vi "Set Values.vi"(0 "image in":refnum<class "MSC Image.lvclass">, 1 "imageData U8":u8[][](array[numeric]), 2 "imageData U16":u16[][](array[numeric]), 3 "imageData Single":sgl[][](array[numeric]), 4 "imageData Double":dbl[][](array[numeric]), 5 "error in (no error)":errorcluster, 9 "imageData BGR":u32[][](array[numeric])) -> (14 "image out":refnum<class "MSC Image.lvclass">, 19 "error out":errorcluster)   [LabVIEW 2014, in "MSC Image.lvclass"]
doc: "Sets the values of the image to the connected array values."
uses:
  MSC Image.lvclass
  controls/Image Type.ctl
  MSC Image.lvclass/MSC Image.ctl
  Dependencies/x86/MSC I Process32.dll
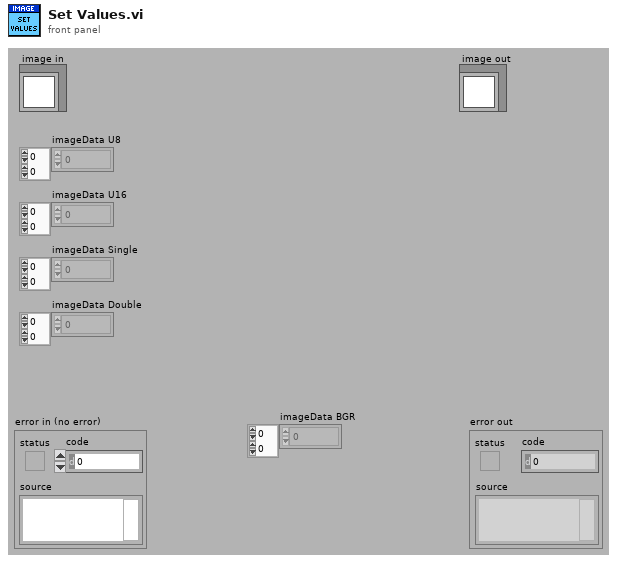
[diagram p1: front panel]
types:
  T1 = typedef "MSC Image.lvclass/Image Type.ctl" = i32
  T2 = typedef "Image.ctl" = cluster{"Pointer":u64, "Size":T3, "Image Type":T4, "Time Stamp":timestamp, "Variant":variant}
  T3 = typedef "Size.ctl" = cluster{"Cols":i32, "Rows":i32}
  T4 = typedef "Image Type.ctl" = i32
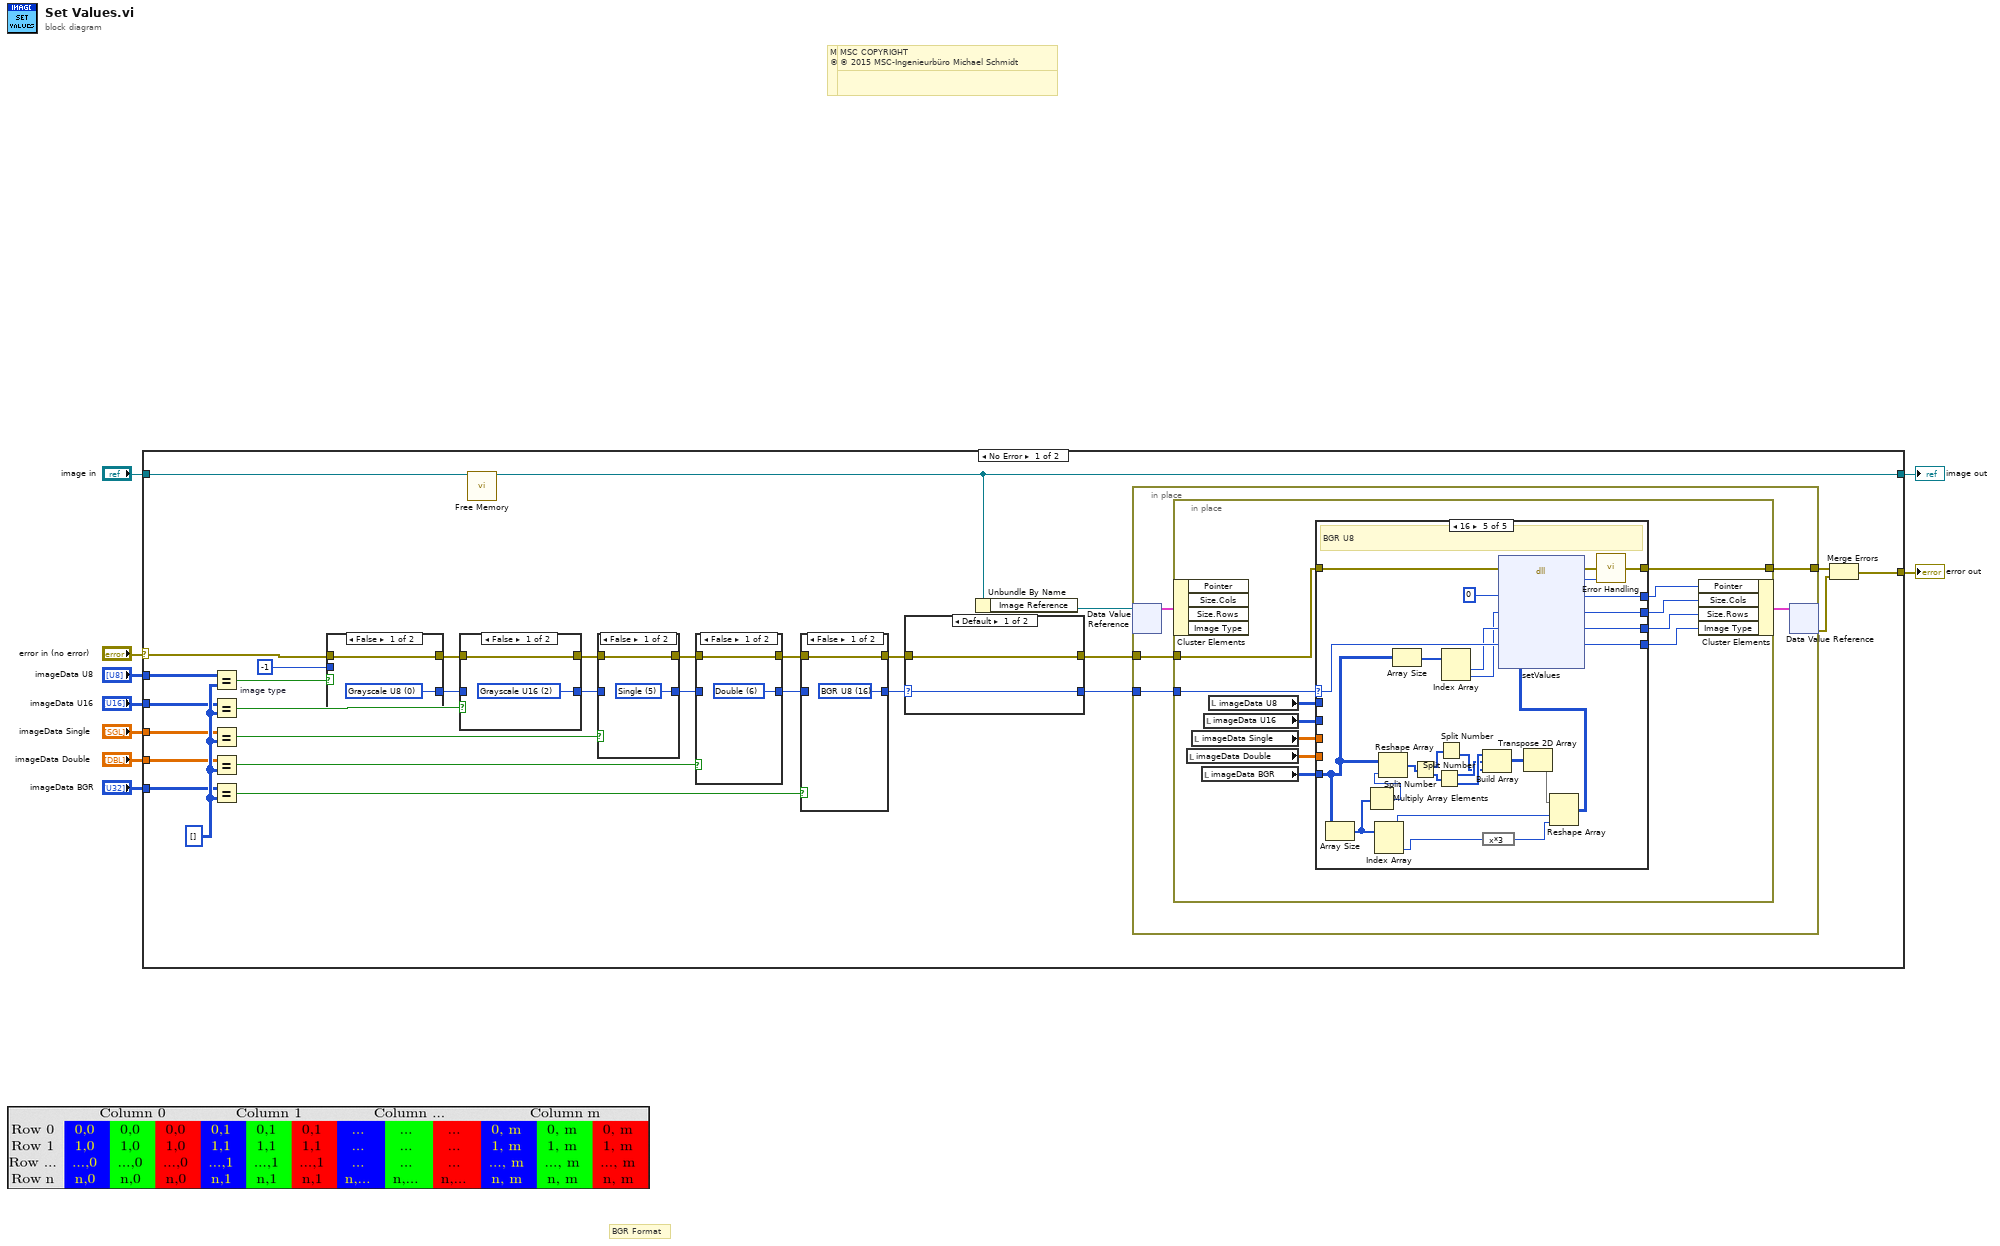
[diagram p0: block diagram]
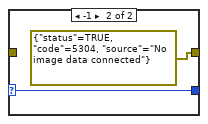
[diagram p7: hidden frame]
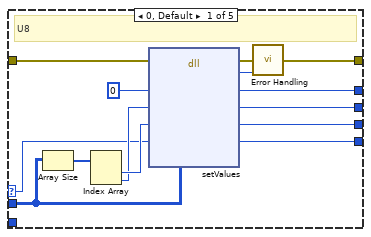
[diagram p8: hidden frame]
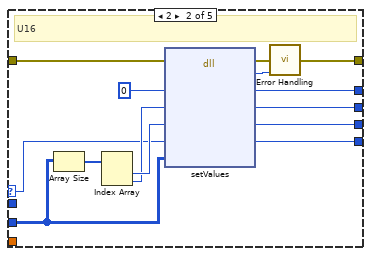
[diagram p9: hidden frame]
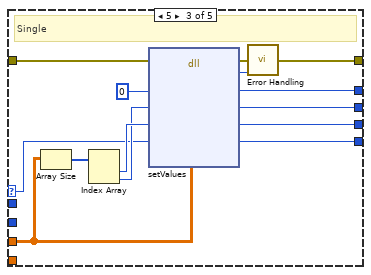
[diagram p10: hidden frame]
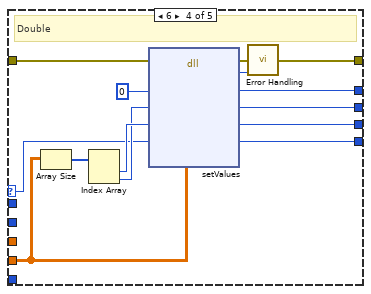
[diagram p11: hidden frame]
diagram:
  # "MSC COPYRIGHT\n© 2016 MSC-Ingenieurbüro Michael Schmidt"
  # "MSC COPYRIGHT\n© 2016 MSC-Ingenieurbüro Michael Schmidt"
  # "MSC COPYRIGHT\n© 2015 MSC-Ingenieurbüro Michael Schmidt"
  # "MSC COPYRIGHT\n© 2015 MSC-Ingenieurbüro Michael Schmidt"
  # "BGR Format"
  n1 = case shown="No Error" "error in (no error)" {
    selector: "error in (no error)" -> [w17 w167]
    tunnel: [w12 w167] -> w8
    tunnel: [w10 w166] -> w6
    tunnel: "image in" -> [w11 w166]
    tunnel: "imageData U8" -> [w18 _]
    tunnel: "imageData U16" -> [w16 _]
    tunnel: "imageData Single" -> [w15 _]
    tunnel: "imageData Double" -> [w14 _]
    tunnel: "imageData BGR" -> [w13 _]
    frame No Error {
      w21 = u32[][] [] ("imageData U8")
      w37 = -1  # image type
      n2 = Equal?(x=w18, y=w21) -> (x = y?=w38:bool)
      n3 = Equal?(x=w16, y=w21) -> (x = y?=w36:bool)
      n4 = Equal?(x=w15, y=w21) -> (x = y?=w20:bool)
      n5 = Equal?(x=w14, y=w21) -> (x = y?=w35:bool)
      n6 = Equal?(x=w13, y=w21) -> (x = y?=w34:bool)
      n7 = case shown="False" w38 {
        tunnel: w17 -> [w58 w59]
        tunnel: w37 -> [_ w60]
        tunnel: [w57 w60] -> w27
        tunnel: [w58 w59] -> w33
        frame False {
          w57 = T1 0 items=["Grayscale U8"=0, "Grayscale U16"=2, "Double"=6, "BGR U8"=16] ("Image.Image Type")
        }
        frame True {
        }
      }
      n8 = case shown="False" w36 {
        tunnel: w33 -> [w54 w55]
        tunnel: w27 -> [_ w56]
        tunnel: [w53 w56] -> w23
        tunnel: [w54 w55] -> w25
        frame False {
          w53 = T1 2 items=["Grayscale U8"=0, "Grayscale U16"=2, "Double"=6, "BGR U8"=16] ("Image.Image Type")
        }
        frame True {
        }
      }
      n9 = call "Free Memory.vi"("image in"=w11) -> ("image out"=w10:refnum<class "MSC Image.lvclass">)  [unwired: 17 in, 1 out]
      n10 = case shown="False" w20 {
        tunnel: w25 -> [w42 w43]
        tunnel: w23 -> [_ w44]
        tunnel: [w41 w44] -> w22
        tunnel: [w42 w43] -> w24
        frame False {
          w41 = T1 5 items=["Grayscale U8"=0, "Grayscale U16"=2, "Single"=5, "Double"=6, "BGR U8"=16] ("Image.Image Type")
        }
        frame True {
        }
      }
      n11 = case shown="False" w35 {
        tunnel: w24 -> [w50 w51]
        tunnel: w22 -> [_ w52]
        tunnel: [w49 w52] -> w26
        tunnel: [w50 w51] -> w32
        frame False {
          w49 = T1 6 items=["Grayscale U8"=0, "Grayscale U16"=2, "Double"=6, "BGR U8"=16] ("Image.Image Type")
        }
        frame True {
        }
      }
      n12 = case shown="False" w34 {
        tunnel: w32 -> [w46 w47]
        tunnel: w26 -> [_ w48]
        tunnel: [w45 w48] -> w31
        tunnel: [w46 w47] -> w30
        frame False {
          w45 = T1 16 items=["Grayscale U8"=0, "Grayscale U16"=2, "Double"=6, "BGR U8"=16] ("Image.Image Type")
        }
        frame True {
        }
      }
      n13 = case shown="Default" w31 {
        selector: w31 -> [w61 w64]
        tunnel: w30 -> [w62 _]
        tunnel: [w62 errorcluster {"status"=TRUE, "code"=5304, "source"="No image data connected"} ("error out")] -> w28
        tunnel: [w61 w64] -> w29
        frame Default {
        }
        frame -1 {
        }
      }
      n14 = Unbundle By Name(w10) -> ("Image Reference"=w19:refnum<data-value>)
      n15 = in-place {
        in-place-border: w28 -> [w67]
        in-place-border: [w66] -> w39
        in-place-border: w29 -> [w65]
        n16 = in-place-dvr #1(w19) -> (w68:T2)  [unwired: 1 out]
        n17 = in-place {
          in-place-border: w67 -> [w79]
          in-place-border: [w78] -> w66
          in-place-border: w65 -> [w75]
          n18 = in-place-cluster #2(w68) -> ()  [unwired: 4 out]
          n19 = local read "imageData Double"() -> (w71:dbl[][])
          n20 = local read "imageData Single"() -> (w72:sgl[][])
          n21 = local read "imageData BGR"() -> (w70:u32[][])
          n22 = local read "imageData U16"() -> (w73:u16[][])
          n23 = local read "imageData U8"() -> (w74:u8[][])
          n24 = case shown="16" w75 {
            selector: w75 -> [w83 w98 w113 w126 w157]
            tunnel: [w95 w109 w123 w137 w165] -> w81
            tunnel: [w94 w108 w122 w136 w164] -> w80
            tunnel: w79 -> [w84 w97 w112 w125 w155]
            tunnel: [w91 w105 w119 w133 w161] -> w78
            tunnel: [w90 w104 w118 w132 w160] -> w76
            tunnel: [w89 w103 w117 w131 w159] -> w77
            tunnel: w74 -> [w87 _ _ _ _]
            tunnel: w73 -> [_ w101 _ _ _]
            tunnel: w70 -> [_ _ _ _ w139]
            tunnel: w71 -> [_ _ _ w129 _]
            tunnel: w72 -> [_ _ w110 _ _]
            frame 0, Default {
              # "U8"
              n25 = Array Size(array=w87) -> (size(s)=w88:i32[])
              n26 = Index Array(array=w88) -> (element #1=w86:i32, element #2=w85:i32)  [unwired: 2 in]
              n27 = dll-call lib="C:/Users/MSC/LabVIEW Projekte/LV 2014/MSC I-Process/user.lib/MSC-I Process/Dependencies/x86/MSC I Process*.dll" fn="setValues"(error in=w84, "pointer"=u64 0, "cols"=w85, "rows"=w86, "type"=w83, "imageData"=w87) -> (error out=w93:errorcluster, "error"=w92:i32, "pointer"=w90:u64, "cols"=w95:i32, "rows"=w94:i32, "type"=w89:i32)  [unwired: 3 in, 1 out]
              n28 = call "Error Handling.vi"("error in (no error)"=w93, "return type"=w92) -> ("error out"=w91:errorcluster)  [unwired: 12 in, 1 out]
            }
            frame 2 {
              # "U16"
              n29 = Array Size(array=w101) -> (size(s)=w102:i32[])
              n30 = Index Array(array=w102) -> (element #1=w100:i32, element #2=w99:i32)  [unwired: 2 in]
              n31 = dll-call lib="C:/Users/MSC/LabVIEW Projekte/LV 2014/MSC I-Process/user.lib/MSC-I Process/Dependencies/x86/MSC I Process*.dll" fn="setValues"(error in=w97, "pointer"=u64 0, "cols"=w99, "rows"=w100, "type"=w98, "imageData"=w101) -> (error out=w107:errorcluster, "error"=w106:i32, "pointer"=w104:u64, "cols"=w109:i32, "rows"=w108:i32, "type"=w103:i32)  [unwired: 3 in, 1 out]
              n32 = call "Error Handling.vi"("error in (no error)"=w107, "return type"=w106) -> ("error out"=w105:errorcluster)  [unwired: 12 in, 1 out]
            }
            frame 5 {
              # "Single"
              n33 = Array Size(array=w110) -> (size(s)=w116:i32[])
              n34 = Index Array(array=w116) -> (element #1=w115:i32, element #2=w114:i32)  [unwired: 2 in]
              n35 = dll-call lib="C:/Users/MSC/LabVIEW Projekte/LV 2014/MSC I-Process/user.lib/MSC-I Process/Dependencies/x86/MSC I Process*.dll" fn="setValues"(error in=w112, "pointer"=u64 0, "cols"=w114, "rows"=w115, "type"=w113, "imageData"=w110) -> (error out=w121:errorcluster, "error"=w120:i32, "pointer"=w118:u64, "cols"=w123:i32, "rows"=w122:i32, "type"=w117:i32)  [unwired: 3 in, 1 out]
              n36 = call "Error Handling.vi"("error in (no error)"=w121, "return type"=w120) -> ("error out"=w119:errorcluster)  [unwired: 12 in, 1 out]
            }
            frame 6 {
              # "Double"
              n37 = Array Size(array=w129) -> (size(s)=w130:i32[])
              n38 = Index Array(array=w130) -> (element #1=w128:i32, element #2=w127:i32)  [unwired: 2 in]
              n39 = dll-call lib="C:/Users/MSC/LabVIEW Projekte/LV 2014/MSC I-Process/user.lib/MSC-I Process/Dependencies/x86/MSC I Process*.dll" fn="setValues"(error in=w125, "pointer"=u64 0, "cols"=w127, "rows"=w128, "type"=w126, "imageData"=w129) -> (error out=w135:errorcluster, "error"=w134:i32, "pointer"=w132:u64, "cols"=w137:i32, "rows"=w136:i32, "type"=w131:i32)  [unwired: 3 in, 1 out]
              n40 = call "Error Handling.vi"("error in (no error)"=w135, "return type"=w134) -> ("error out"=w133:errorcluster)  [unwired: 12 in, 1 out]
            }
            frame 16 {
              # "BGR U8"
              n41 = Array Size(array=w139) -> (size(s)=w152:i32[])
              n42 = Multiply Array Elements(1:w152) -> (0:w151:i32)
              n43 = Index Array(array=w152) -> (element #1=w141:i32, element #2=w142:i32)  [unwired: 2 in]
              n44 = Reshape Array(w139, w151) -> (w150:u32[])
              n45 = Array Size(array=w139) -> (size(s)=w158:i32[])
              n46 = Split Number(x=w150) -> (hi(x)=w149:u16[], lo(x)=w148:u16[])
              n47 = Split Number(x=w148) -> (hi(x)=w146:u8[], lo(x)=w147:u8[])
              n48 = Split Number(x=w149) -> (lo(x)=w145:u8[])  [unwired: 1 out]
              n49 = Index Array(array=w158) -> (element #1=w156:i32, element #2=w153:i32)  [unwired: 2 in]
              n50 = Build Array(w147, w146, w145) -> (w144:u8[][])
              n51 = expression code="x*3"(w142) -> (w140:i32)
              n52 = Transpose 2D Array(2D array=w144) -> (transposed array=w143:u8[][])
              n53 = Reshape Array(w143, w141, w140) -> (w138:u8[][])
              n54 = dll-call lib="C:/Users/MSC/LabVIEW Projekte/LV 2014/MSC I-Process/user.lib/MSC-I Process/Dependencies/x86/MSC I Process*.dll" fn="setValues"(error in=w155, "pointer"=u64 0, "cols"=w153, "rows"=w156, "type"=w157, "imageData"=w138) -> (error out=w163:errorcluster, "error"=w162:i32, "pointer"=w160:u64, "cols"=w165:i32, "rows"=w164:i32, "type"=w159:i32)  [unwired: 3 in, 1 out]
              n55 = call "Error Handling.vi"("error in (no error)"=w163, "return type"=w162) -> ("error out"=w161:errorcluster)  [unwired: 12 in, 1 out]
            }
          }
          n56 = in-place-cluster #2("Pointer"=w76, "Size.Cols"=w81, "Size.Rows"=w80, "Image Type"=w77) -> (w69:T2)
        }
        n57 = in-place-dvr #1(w69) -> (w40:errorcluster)  [unwired: 1 out]
      }
      n58 = Merge Errors(w39, w40) -> (w12:errorcluster)
    }
    frame Error {
    }
  }
  "error out" <- w8
  "image out" <- w6
